vi "CH1_Tx.vi"() -> ()   [LabVIEW 2018]
uses:
  Stream/Stream.lvclass
  RxTx/RxTx.lvclass
  Interface/Interface.lvclass
panel:
  out "value":T1
  in  "RxTx.lvclass":refnum<class "RxTx.lvclass">
  in  "Stream.lvclass":refnum<class "Stream.lvclass">
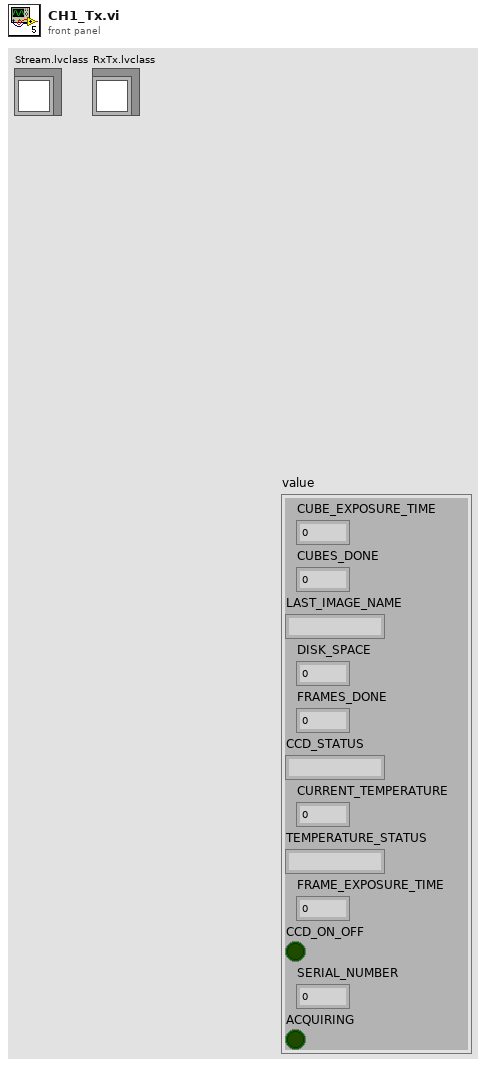
[diagram p1: front panel]
types:
  T1 = cluster{"CUBE_EXPOSURE_TIME":sgl, "CUBES_DONE":u16, "LAST_IMAGE_NAME":string, "DISK_SPACE":u16, "FRAMES_DONE":u16, "CCD_STATUS":string, "CURRENT_TEMPERATURE":i16, "TEMPERATURE_STATUS":string, "FRAME_EXPOSURE_TIME":u16, "CCD_ON_OFF":bool, "SERIAL_NUMBER":u16, "ACQUIRING":bool}
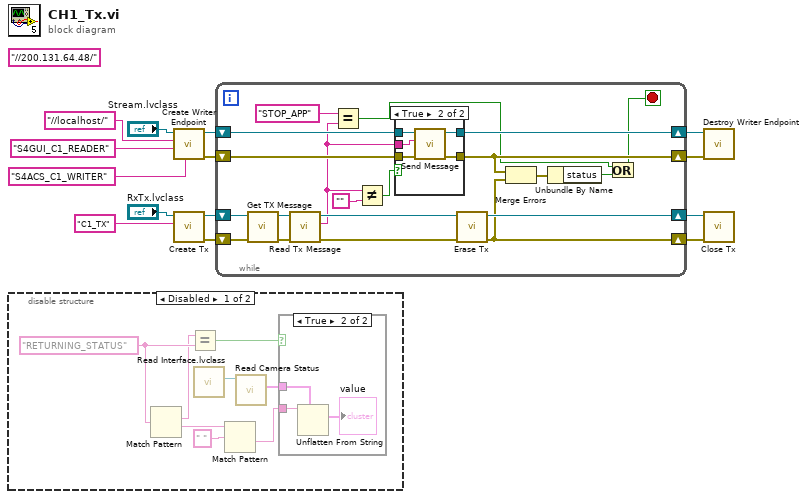
[diagram p0: block diagram]
diagram:
  (unwired) "//200.131.64.48/" ("Reader Name")
  n1 = disable-structure shown="Disabled" {
    frame Disabled {
      w19 = "RETURNING_STATUS" ("regular expression")
      n2 = Match Pattern(regular expression=w19) -> (match substring=w18:string, after substring=w16:string)  [unwired: 2 in, 2 out]
      n3 = Equal?(x=w18, y=w19) -> (x = y?=w20:bool)
      n4 = call "Read Interface.lvclass.vi"() -> ("Interface.lvclass"=w23:refnum<class "Interface.lvclass">, "RxTx in"=w21:refnum<class "RxTx.lvclass">)  [unwired: 8 in, 2 out]
      n5 = Match Pattern(string=w16, regular expression=" ") -> (after substring=w17:string)  [unwired: 1 in, 3 out]
      n6 = call "Read Camera Status.vi"("Interface in"=w23) -> ("Camera Status"=w22:T1)  [unwired: 8 in, 2 out]
      n7 = case shown="True" w20 {
        tunnel: w22 -> [_ w26]
        tunnel: w17 -> [_ w24]
        frame False {
        }
        frame True {
          n8 = Unflatten From String(type=w26, binary string=w24) -> (value=→"value":T1)  [unwired: 3 in, 2 out]
        }
      }
    }
    frame Enabled {
    }
  }
  n9 = call "Create Writer Endpoint.vi"("writer name"="S4ACS_C1_WRITER" ("reader name"), "reader name"="S4GUI_C1_READER", "IP"="//localhost/" ("Reader Name"), "Stream in"="Stream.lvclass") -> ("error out"=w6:errorcluster, "Stream out"=w8:refnum<class "Stream.lvclass">)  [unwired: 6 in]
  n10 = call "Create Tx.vi"("Writer Name"="C1_TX" ("Reader Name"), "RxTx in"="RxTx.lvclass") -> ("error out"=w12:errorcluster, "RxTx out"=w13:refnum<class "RxTx.lvclass">)  [unwired: 8 in]
  n11 = while {
    shift-right: [w39] -> w4
    shift-left: w6 -> [w41]
    shift-right: [w40] -> w14
    shift-left: w8 -> [w42]
    shift-right: [w34] -> w9
    shift-left: w12 -> [w43]
    shift-right: [w36] -> w10
    shift-left: w13 -> [w44]
    stop <- w31 stop-if-true
    n12 = call "Get TX Message.vi"("error in (no error)"=w43, "RxTx in"=w44) -> ("error out"=w45:errorcluster, "RxTx out"=w28:refnum<class "RxTx.lvclass">)  [unwired: 8 in]
    n13 = call "Read Tx Message.vi"("error in (no error)"=w45, "RxTx in"=w28) -> ("error out"=w35:errorcluster, "Tx Message"=w27:string, "RxTx out"=w37:refnum<class "RxTx.lvclass">)  [unwired: 7 in]
    n14 = Equal?(x="STOP_APP", y=w27) -> (x = y?=w33:bool)
    n15 = Not Equal?(x=w27, y="") -> (x != y?=w29:bool)
    n16 = case shown="True" w29 {
      tunnel: w42 -> [w48 w53]
      tunnel: w41 -> [w47 w52]
      tunnel: [w48 w51] -> w40
      tunnel: w27 -> [_ w50]
      tunnel: [w47 w49] -> w39
      frame False {
      }
      frame True {
        n17 = call "Send Message.vi"("error in (no error)"=w52, "Message"=w50, "Stream in"=w53) -> ("error out"=w49:errorcluster, "Stream out"=w51:refnum<class "Stream.lvclass">)  [unwired: 7 in]
      }
    }
    n18 = call "Erase Tx.vi"("error in (no error)"=w35, "RxTx in"=w37) -> ("error out"=w34:errorcluster, "RxTx out"=w36:refnum<class "RxTx.lvclass">)  [unwired: 8 in]
    n19 = Merge Errors(w39, w34) -> (w46:errorcluster)
    n20 = Unbundle By Name(w46) -> ("status"=w32:bool)
    n21 = Or(x=w33, y=w32) -> (x .or. y?=w31:bool)
  }
  n22 = call "Destroy Writer Endpoint.vi"("error in (no error)"=w4, "Stream in"=w14) -> ()  [unwired: 8 in, 2 out]
  n23 = call "Close Tx.vi"("error in (no error)"=w9, "RxTx in"=w10) -> ()  [unwired: 8 in, 2 out]
